vi "Add coreConfiguration.vi"(6 "core builtInTest configuration (default)":T4, 7 "core sequentialLog configuration (default)":T2={"perChannelStreaming (T)"=TRUE, "useDMA (T)"=TRUE}, 8 "error in":errorcluster, 9 "core timing configuration (default)":T3={"driftMax"=425000000, "delayComp"=0, "irigControlVal"=[0, 0, 0, 0], "irigYears"=2000, "irigType"=1, "jumpThreshPPT"=425000000, "jumpThreshNS"=200000, "timerRollover"=0, "timeSourceSelect"=0, "timeSyncSelect"=0, "timeEnableUserInputThresh"=FALSE, "timeInputThreshVal"=[0, 0], "driftSyncSelect"=0, "driftEnableUserInputThresh"=FALSE, "driftInputThreshVal"=[0, 0], "resolution"=0, "timerValue"=0} {"resolution" items=["Item1NS", "Item1US"]; "driftSyncSelect" items=["None", "PPS0", "PPS1", "PWMIRIG0", "PWMIRIG1", "AMIRIG", "Item10MHZ", "HOST"]; "timeSyncSelect" items=["None", "PPS0", "PPS1", "PWMIRIG0", "PWMIRIG1", "AMIRIG"]; "timeSourceSelect" items=["None", "PPS0", "PPS1", "PWMIRIG0", "PWMIRIG1", "AMIRIG", "Item10MHZ"]; "irigType" items=["A", "B"]}, 10 "core generic configuration (default)":T1, 11 "xml ref in":refnum<k24>) -> (0 "error out":errorcluster, 2 "new coreConfiguration out":refnum<k24>, 3 "xml ref out":refnum<k24>)   [LabVIEW 2020, in "Ballard_1553_Hardware_ni.lvlib"]
uses:
  Ballard_1553_Hardware_ni.lvlib
  C:/Users/Administrator/Desktop/GIT/Ballard-MIL-STD-1553-Custom-Device/Source/System Explorer/SubVIs/Parse XML Ballard/1.2/BTIXML_SerDes.dll
  Ballard-MIL-STD-1553-Custom-Device/Source/System Explorer/SubVIs/Parse XML Ballard/1.2/BTIXML_SerDes.dll
  _typedefs/core_builtInTests_type.ctl
  _typedefs/core_timing_type.ctl
  _typedefs/core_sequentialLog_type.ctl
  _typedefs/core_generic_type.ctl
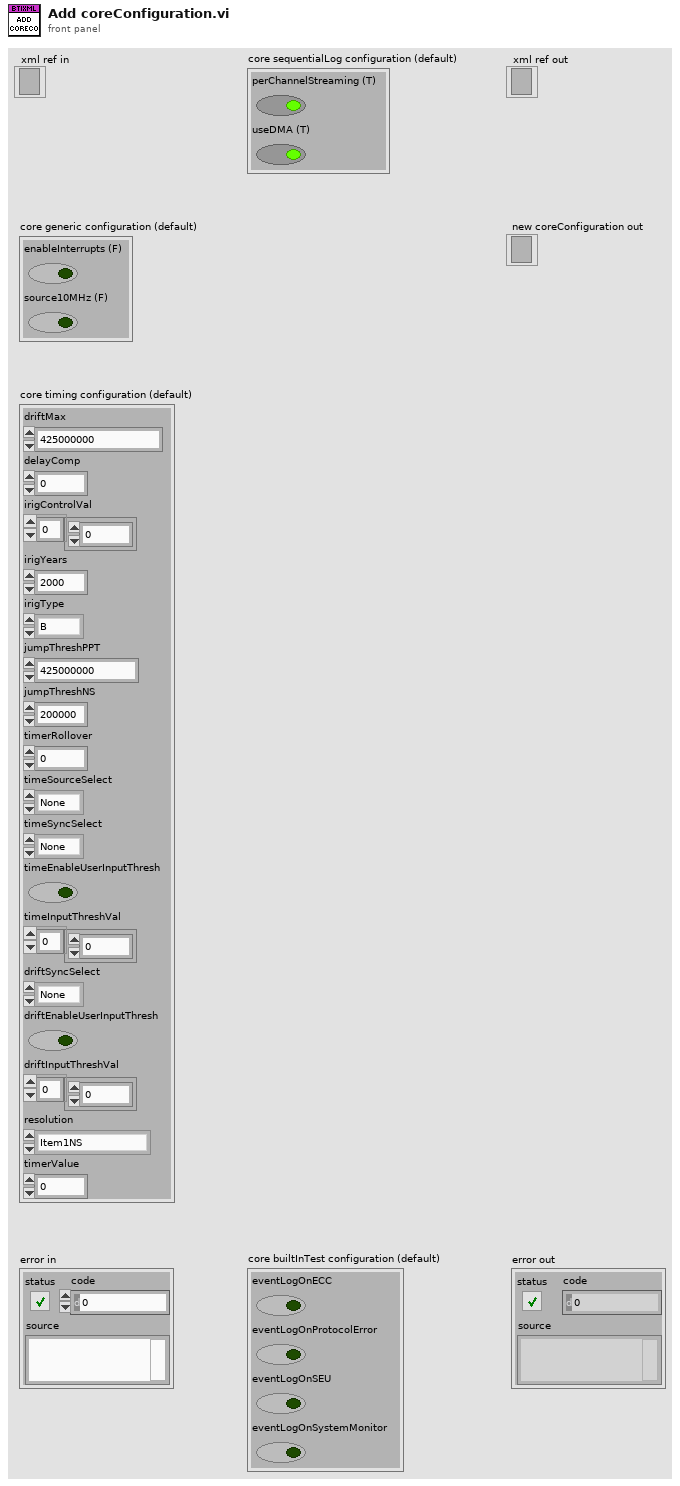
[diagram p1: front panel]
types:
  T1 = typedef "Ballard_1553_Hardware_ni.lvlib/core_generic_type.ctl" = cluster{"enableInterrupts (F)":bool, "source10MHz (F)":bool}
  T2 = typedef "Ballard_1553_Hardware_ni.lvlib/core_sequentialLog_type.ctl" = cluster{"perChannelStreaming (T)":bool, "useDMA (T)":bool}
  T3 = typedef "Ballard_1553_Hardware_ni.lvlib/core_timing_type.ctl" = cluster{"driftMax":u32, "delayComp":i32, "irigControlVal":u8[], "irigYears":u32, "irigType":i32, "jumpThreshPPT":u32, "jumpThreshNS":u32, "timerRollover":u64, "timeSourceSelect":i32, "timeSyncSelect":i32, "timeEnableUserInputThresh":bool, "timeInputThreshVal":u8[], "driftSyncSelect":i32, "driftEnableUserInputThresh":bool, "driftInputThreshVal":u8[], "resolution":i32, "timerValue":u64}
  T4 = typedef "Ballard_1553_Hardware_ni.lvlib/core_builtInTests_type.ctl" = cluster{"eventLogOnECC":bool, "eventLogOnProtocolError":bool, "eventLogOnSEU":bool, "eventLogOnSystemMonitor":bool}
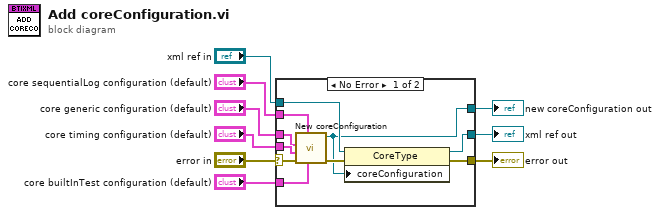
[diagram p0: block diagram]
diagram:
  n1 = case shown="No Error" "error in" {
    selector: "error in" -> [w16 w20]
    tunnel: [w19 w20] -> w9
    tunnel: [w18 w21] -> w8
    tunnel: "xml ref in" -> [w17 w21]
    tunnel: [w14 _] -> w5
    tunnel: "core sequentialLog configuration (default)" -> [w13 _]
    tunnel: "core timing configuration (default)" -> [w12 _]
    tunnel: "core generic configuration (default)" -> [w11 _]
    tunnel: "core builtInTest configuration (default)" -> [w10 _]
    frame No Error {
      n2 = call "New coreConfiguration.vi"("core builtInTest configuration (default)"=w10, "core sequentialLog configuration (default)"=w13, "error in"=w16, "core timing configuration (default)"=w12, "core generic configuration (default)"=w11) -> ("error out"=w15:errorcluster, "new CoreConfigurationType"=w14:refnum<k24>)  [unwired: 5 in]
      n3 = property class="CoreType"(reference=w17, error in=w15, "coreConfiguration"=w14) -> (reference out=w18:refnum<k24>, error out=w19:errorcluster)
    }
    frame Error {
    }
  }
  "error out" <- w9
  "xml ref out" <- w8
  "new coreConfiguration out" <- w5
